vi "Create request.vi"(8 "error in (no error)":errorcluster, 10 "Options":string="{}", 11 "Topic":string) -> (0 "error out":errorcluster, 2 "notifier out":refnum<notifier>, 3 "Subscribe JSON out":refnum<class "Subscribe JSON.lvclass">)   [LabVIEW 2020, in "wamplv.lvlib" / "Subscribe JSON.lvclass"]
uses:
  Subscribe JSON.lvclass
  Subscribe result (JSON).ctl
  wamplv.lvlib
  WAMP Client/Private/TypeDef/SUBSCRIBE Request Data (JSON).ctl
  Message loop classes/Subscription details/SubscriptionDetails JSON/SubscriptionDetails JSON.lvclass
  Message loop classes/ErrorOrSuccess JSON/ErrorOrSuccess JSON.lvclass
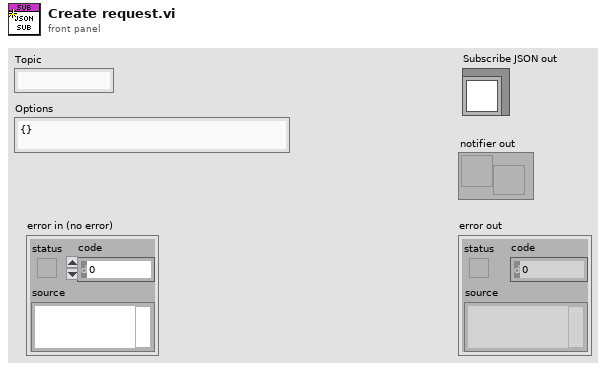
[diagram p1: front panel]
types:
  T1 = typedef "wamplv.lvlib/SUBSCRIBE Request Data (JSON).ctl" = cluster{"Topic":string, "Options":string, "Subscribe result notifer":refnum<notifier>}
  T2 = typedef "wamplv.lvlib/Subscribe result (JSON).ctl" = cluster{"SubscriptionDetails JSON":refnum<class "SubscriptionDetails JSON.lvclass">, "ErrorOrSuccess JSON":refnum<class "ErrorOrSuccess JSON.lvclass">}
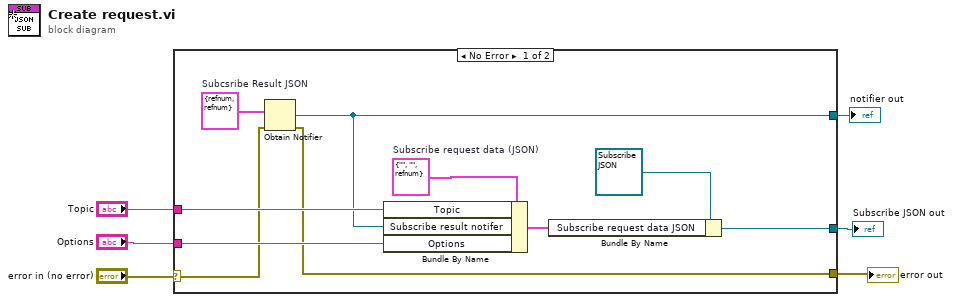
[diagram p0: block diagram]
diagram:
  n1 = case shown="No Error" "error in (no error)" {
    selector: "error in (no error)" -> [w9 w17]
    tunnel: [w8 w17] -> w2
    tunnel: "Topic" -> [w16 _]
    tunnel: [w15 _] -> w5
    tunnel: "Options" -> [w14 _]
    tunnel: [w10 _] -> w1
    frame No Error {
      w7 = T1 {"Topic"="", "Options"="", "Subscribe result notifer"=refnum}  # Subscribe request data (JSON)
      w13 = T2 {"SubscriptionDetails JSON"=refnum, "ErrorOrSuccess JSON"=refnum}  # Subcsribe Result JSON
      n2 = Obtain Notifier(notification data type=w13, error in (no error)=w9) -> (notifier out=w15:refnum<notifier>, error out=w8:errorcluster)  [unwired: 2 in, 1 out]
      n3 = Bundle By Name(cluster=w7, "Topic"=w16, "Subscribe result notifer"=w15, "Options"=w14) -> (w11:T1)
      n4 = Bundle By Name(cluster=refnum<class "Subscribe JSON.lvclass"> refnum ("wamplv.lvlib:Subscribe JSON.lvclass"), "Subscribe request data JSON"=w11) -> (w10:refnum<class "Subscribe JSON.lvclass">)
    }
    frame Error {
    }
  }
  "error out" <- w2
  "Subscribe JSON out" <- w1
  "notifier out" <- w5
